vi "Read Actor Name.vi"(8 "error in (no error)":errorcluster, 11 "CS++GUIActor in":refnum<class "CS++GUIActor.lvclass">) -> (0 "error out":errorcluster, 2 "Actor Name":string, 3 "CS++GUIActor out":refnum<class "CS++GUIActor.lvclass">)   [LabVIEW 2013, in "CS++GUIActor.lvlib" / "CS++GUIActor.lvclass"]
doc: "Read assoziated actor name."
uses:
  CS++GUIActor.lvclass
  CS++GUIActor.lvclass/CS++GUIActor.ctl
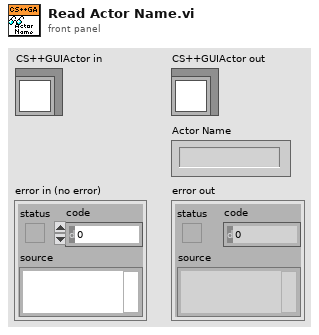
[diagram p1: front panel]
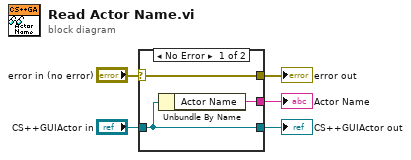
[diagram p0: block diagram]
diagram:
  n1 = case shown="No Error" "error in (no error)" {
    selector: "error in (no error)" -> [w8 w9]
    tunnel: [w8 w9] -> w4
    tunnel: [w7 w10] -> w2
    tunnel: "CS++GUIActor in" -> [w7 w10]
    tunnel: [w6 _] -> w1
    frame No Error {
      n2 = Unbundle By Name(w7) -> ("Actor Name"=w6:string)
    }
    frame Error {
    }
  }
  "error out" <- w4
  "CS++GUIActor out" <- w2
  "Actor Name" <- w1
